vi "UsrProfiles-Export profile.vi"   [LabVIEW 2013]
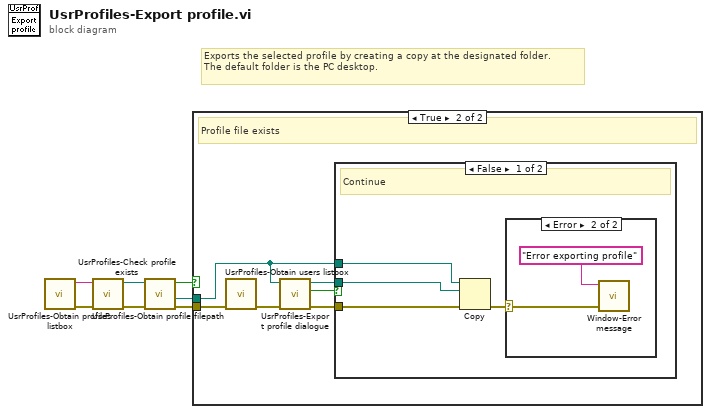
[diagram p0: block diagram]
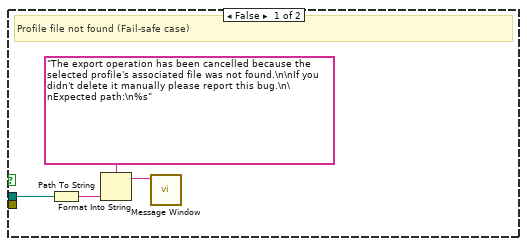
[diagram p2: hidden frame]
diagram:
  # "Exports the selected profile by creating a copy at the designated folder.\nThe default folder is the PC desktop."
  n1 = call "UsrProfiles-Obtain profiles listbox.vi"() -> ("error out"=w6:errorcluster, "Selected profile's name"=w7:string)  [unwired: 8 in, 2 out]
  n2 = call "UsrProfiles-Obtain profile filepath.vi"("error in"=w6, "Profile name"=w7) -> ("error out"=w5:errorcluster, "Profile filepath"=w1:path)  [unwired: 8 in]
  n3 = call "UsrProfiles-Check profile exists.vi"("error in"=w5, "Profile file path"=w1) -> ("error out"=w4:errorcluster, "Profile's file path"=w3:path, "Profile file exists"=w2:bool)  [unwired: 7 in]
  n4 = case shown="True" w2 {
    tunnel: w4 -> [_ w17]
    tunnel: w3 -> [w8 w12]
    frame False {
      # "Profile file not found (Fail-safe case)"
      n5 = Path To String(path=w8) -> (string=w11:string)
      n6 = Format Into String(format string="The export operation has been cancelled because the selected profile's associated file was not found.\n\nIf you didn't delete it manually please report this bug.\n\nExpected path:\n%s", w11) -> (resulting string=w9:string)  [unwired: 2 in, 1 out]
      n7 = call "Message Window.vi"("Message string"=w9) -> ()  [unwired: 10 in, 1 out]
    }
    frame True {
      # "Profile file exists"
      n8 = call "UsrProfiles-Obtain users listbox.vi"("error in (no error)"=w17) -> ("error out"=w14:errorcluster)  [unwired: 7 in, 3 out]
      n9 = call "UsrProfiles-Export profile dialogue.vi"("error in (no error)"=w14, "Profile's file path"=w12) -> ("error out"=w13:errorcluster, "cancelled"=w16:bool, "selected path"=w15:path)  [unwired: 7 in]
      n10 = case shown="False" w16 {
        tunnel: w12 -> [w19 _]
        tunnel: w15 -> [w21 _]
        tunnel: w13 -> [w20 _]
        frame False {
          # "Continue"
          n11 = Copy(8:w20, 10:w21, 11:w19) -> (0:w18:errorcluster)  [unwired: 2 in, 2 out]
          n12 = case shown="Error" w18 {
            selector: w18 -> [_ w23]
            frame No Error {
            }
            frame Error {
              n13 = call "Window-Error message.vi"("error in (no error)"=w23, "Message"="Error exporting profile") -> ()  [unwired: 9 in, 1 out]
            }
          }
        }
        frame True {
          # "Cancelled"
        }
      }
    }
  }
